vi "lift height calculation.vi"(10 "intial position":dbl format="%#_13g", 11 "curreent position":dbl format="%#_13g") -> (3 "real world height":dbl format="%#_13g")   [LabVIEW 2014]
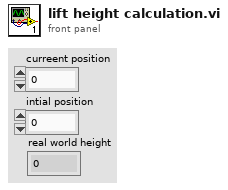
[diagram p1: front panel]
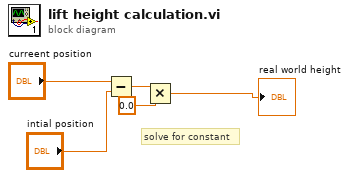
[diagram p0: block diagram]
diagram:
  # "solve for constant"
  n1 = Subtract(x="curreent position", y="intial position") -> (x-y=w3:dbl)
  n2 = Multiply(x=w3, y=0.0) -> (x*y=→"real world height":dbl)
